vi "cluster_v9.vi"() -> ()   [LabVIEW 2009]
panel:
  out "Mixed Signal Graph":cluster{dbl[], dbl[], dbl[], dbl[], dbl[]}(graph)={[0.0, 0.004230646640570575, 0.00846129328114115, 0.012691939921711725, 0.0169225865622823, 0.021153233202852877, 0.02538387984342345, 0.029614526483994028, 0.0338451731245646, 0.038075819765135174, 0.042306466405705755, 0.04653711304627633, 0.0507677596868469, 0.054998406327417475, 0.059229052967988055, 0.06345969960855863, 0.0676903462491292, 0.07192099288969978, 0.07615163953027035, 0.08038228617084092, 0.08461293281141151, 0.08884357945198207, 0.09307422609255266, 0.09730487273312322, 0.1015355193736938, 0.10576616601426438, 0.10999681265483495, 0.11422745929540552, 0.11845810593597611, 0.12268875257654667, 0.12691939921711726, 0.13115004585768783, 0.1353806924982584, 0.13961133913882898, 0.14384198577939955, 0.14807263241997012, 0.1523032790605407, 0.15653392570111127, 0.16076457234168184, 0.16499521898225245, 0.16922586562282302, 0.17345651226339356, 0.17768715890396414, 0.18191780554453474, 0.1861484521851053, 0.19037909882567586, 0.19460974546624643, 0.19884039210681703, 0.2030710387473876, 0.2073016853879582, 0.21153233202852875, 0.21576297866909933, 0.2199936253096699, 0.2242242719502405, 0.22845491859081105, 0.23268556523138162, 0.23691621187195222, 0.2411468585125228, 0.24537750515309334, 0.2496081517936639, 0.2538387984342345, 0.2580694450748051, 0.26230009171537566, 0.2665307383559462, 0.2707613849965168, 0.2749920316370874, 0.27922267827765795, 0.2834533249182285, 0.2876839715587991, 0.2919146181993697, 0.29614526483994025, 0.3003759114805108, 0.3046065581210814, 0.308837204761652, 0.31306785140222254, 0.3172984980427931, 0.3215291446833637, 0.3257597913239343, 0.3299904379645049, 0.33422108460507544, 0.33845173124564604, 0.34268237788621664, 0.34691302452678713, 0.35114367116735773, 0.3553743178079283, 0.3596049644484989, 0.3638356110890695, 0.36806625772964, 0.3722969043702106, 0.3765275510107812, 0.3807581976513517, 0.3849888442919223, 0.38921949093249286, 0.39345013757306346, 0.39768078421363406, 0.40191143085420467, 0.4061420774947752, 0.4103727241353458, 0.4146033707759164, 0.4188340174164869, 0.4230646640570575, 0.42729531069762805, 0.43152595733819865, 0.43575660397876925, 0.4399872506193398, 0.4442178972599104, 0.448448543900481, 0.4526791905410515, 0.4569098371816221, 0.46114048382219264, 0.46537113046276324, 0.46960177710333384, 0.47383242374390444, 0.478063070384475, 0.4822937170250456, 0.4865243636656162, 0.4907550103061867, 0.4949856569467573, 0.4992163035873278, 0.5034469502278984], [0.0, 0.4105568446600889, 0.7487202054388066, 0.9548617406674794, 0.9926325157175458, 0.8553724102418765, 0.5672844971219748, 0.1791673148942777, -0.24054243798854055, -0.6178373454393544, -0.8861890005972879, -0.998278959074209, -0.9343423997307195, -0.7056532553692195, -0.35253628028746176, 0.06274341320109471, 0.4669595613333527, 0.7888367351766151, 0.9716183362245395, 0.9830744867844777, 0.8211851239548108, 0.5144961972940673, 0.11708616185075667, -0.30096967521764056, -0.6659555327812795, -0.9135134586098452, -0.9999915663780399, -0.9101411722988674, -0.6598055953672661, -0.29312650509683696, 0.12523957857763632, 0.5215221687456819, 0.8258447606627524, 0.9845461550595324, 0.9696425368160321, 0.7837618607724106, 0.45968046448105704, 0.05454361696822202, -0.3602109059217929, -0.7114494437517302, -0.9372381090279818, -0.9977635888978398, -0.882353426164791, -0.6113578935480203, -0.23256163031875554, 0.1872422226143023, 0.5740296565032156, 0.8595984474051875, 0.9935942535766267, 0.9523895959962669, 0.743250091479855, 0.40305330654732185, -0.008213863474088874, -0.4180326830398945, -0.7541398042254394, -0.9572694620667934, -0.99160380624181, -0.8510886622215772, -0.560501063798189, -0.17108031899001463, 0.24850701657486107, 0.6242751126536321, 0.8899647850177782, 0.99872697667578, 0.931383651574637, 0.6998094574851441, 0.3448378694917055, -0.07093897621799697, -0.4742071530352126, -0.793858387798745, -0.9735285818155787, -0.9815364917604706, -0.816470082961343, -0.507435513457404, -0.10892484547378199, 0.30879253930837325, 0.6720605390471127, 0.9168241113633988, 0.9999240982558683, 0.9067074799542068, 0.6536111417333007, 0.28526355811438003, -0.13338454555406226, -0.5285129537791516, -0.8304486787055756, -0.9859513972941013, -0.9676013168946559, -0.7786341069812652, -0.4523703535894608, -0.04634014074889865, 0.36786122859775133, 0.71719763157143, 0.940070584096705, 0.9971809009180234, 0.8784583205014747, 0.6048371941397673, 0.22456513202015538, -0.19530449734663968, -0.5807360868548394, -0.8637664885863127, -0.9944889549318572, -0.9498531948455234, -0.7377298314100129, -0.3955225749554867, 0.016427172769559645, 0.4254803173017054, 0.7595085221865201, 0.9596125977483974, 0.9905081945551012, 0.8467474923631642, 0.5536798142012235, 0.16298178052054185, -0.2564548287180254, -0.6306707608431243, -0.8936805246790326, -0.9991076114753917, -0.9283620641825999, -0.6939184443729015, -0.3371161929362305, 0.07912975307502212], [0.0, 0.0, 0.0, 0.0, 0.0, 0.0, 0.0, 0.0, 0.0, 0.0, 0.0, 0.0, 0.0, 0.0, 0.0, 0.0, 0.0, 0.0, 0.0, 0.0, 0.0, 0.0, 0.0, 0.0, 0.0, 0.0, 0.0, 0.0, 0.0, 0.0, 0.0, 0.0, 0.0, 0.0, 0.0, 0.0, 0.0, 0.0, 0.0, 0.0, 0.0, 0.0, 0.0, 0.0, 0.0, 0.0, 0.0, 0.0, 0.0, 0.0, 0.0, 0.0, 0.0, 0.0, 0.0, 0.0, 0.0, 0.0, 0.0, 0.0, 0.0, 0.0, 0.0, 0.0, 0.0, 0.0, 0.0, 0.0, 0.0, 0.0, 0.0, 0.0, 0.0, 0.0, 0.0, 0.0, 0.0, 0.0, 0.0, 0.0, 0.0, 0.0, 0.0, 0.0, 0.0, 0.0, 0.0, 0.0, 0.0, 0.0, 0.0, 0.0, 0.0, 0.0, 0.0, 0.0, 0.0, 0.0, 0.0, 0.0, 0.0, 0.0, 0.0, 0.0, 0.0, 0.0, 0.0, 0.0, 0.0, 0.0, 0.0, 0.0, 0.0, 0.0, 0.0, 0.0, 0.0, 0.0, 0.0, 0.0], [1.0, 0.9982936638442269, 0.9931804785430605, 0.9846778937224019, 0.9728149259180452, 0.957632059551749, 0.9391811087711717, 0.9175250406251635, 0.8927377601778635, 0.8649038582949328, 0.8341183229626493, 0.8004862151250378, 0.7641223101452946, 0.7251507061150838, 0.683704400348416, 0.6399248355053966, 0.5939614168947772, 0.5459710026025942, 0.49611736818692226, 0.44457064776556143, 0.39150675340404506, 0.33710677478540313, 0.2815563612104166, 0.2250450880373876, 0.16776580972356367, 0.10991400167607222, 0.051687093158409365, -0.006716206470939284, -0.06509658588842593, -0.12325481198967517, -0.1809924098067822, -0.2381123398383418, -0.29441967048069734, -0.3497222432656289, -0.40383132863423615, -0.45656227000907845, -0.5077351139665637, -0.5571752243590158, -0.6047138782906183, -0.6501888419133702, -0.6934449240780485, -0.7343345059507433, -0.772718044787567, -0.8084645501483116, -0.8414520309238988, -0.8715679116520576, -0.898709416700489, -0.9227839210064208, -0.943709266175594, -0.96141404086194, -0.9758378244711048, -0.9869313933561374, -0.9946568888016678, -0.998987946223296, -0.9999097851412794, -0.997419259621467, -0.9915248690113416, -0.9822467289345315, -0.9696165026427797, -0.9536772929596405, -0.9344834951846677, -0.9121006114600809, -0.88660502723342, -0.8580837505790422, -0.8266341152680752, -0.7923634486001533, -0.7553887051305126, -0.7158360675424179, -0.6738405160270151, -0.6295453676401688, -0.5831017872083147, -0.5346682714524423, -0.48441010809072127, -0.43249881176568583, -0.379111538720961, -0.3244304822250554, -0.2686422508054387, -0.21193723141478688, -0.15450893970270088, -0.09655335961020424, -0.03826827454077909, 0.020147407609582023, 0.07849433325984448, 0.1365733834723778, 0.19418635348064073, 0.2511366290970993, 0.30722985769302397, 0.36227461146031936, 0.41608304069190793, 0.46847151485122324, 0.5192612492430576, 0.5682789151471406, 0.6153572313322662, 0.6603355349323142, 0.7030603297359688, 0.7433858100189867, 0.7811743581313565, 0.8162970141412415, 0.8486339159329682, 0.878074708257152, 0.9045189193369975, 0.9278763037455517, 0.9480671503837738, 0.9650225545083945, 0.9786846528812267, 0.9890068212374359, 0.9959538333988778, 0.9995019814895009, 0.9996391568425592, 0.9963648913235233, 0.989690358927671, 0.9796383376469019, 0.9662431317359161, 0.9495504546430333, 0.929617273005174, 0.9065116122393948, 0.8803123243944311, 0.8511088190544934, 0.8190007582136563, 0.7840977161621274], [0.0, 0.0005842639199106157, 0.0011685278398212314, 0.0017527917597318472, 0.0023370556796424627, 0.002921319599553078, 0.0035055835194636943, 0.004089847439374309, 0.0046741113592849255, 0.005258375279195541, 0.005842639199106156, 0.0064269031190167724, 0.007011167038927389, 0.007595430958838004, 0.008179694878748619, 0.008763958798659235, 0.009348222718569851, 0.009932486638480467, 0.010516750558391082, 0.011101014478301698, 0.011685278398212312, 0.01226954231812293, 0.012853806238033545, 0.01343807015794416, 0.014022334077854777, 0.014606597997765392, 0.015190861917676008, 0.015775125837586623, 0.016359389757497237, 0.016943653677407855, 0.01752791759731847, 0.018112181517229087, 0.018696445437139702, 0.019280709357050316, 0.019864973276960934, 0.02044923719687155, 0.021033501116782163, 0.02161776503669278, 0.022202028956603396, 0.02278629287651401, 0.023370556796424625, 0.023954820716335243, 0.02453908463624586, 0.025123348556156472, 0.02570761247606709, 0.026291876395977708, 0.02687614031588832, 0.027460404235798937, 0.028044668155709555, 0.028628932075620166, 0.029213195995530784, 0.0297974599154414, 0.030381723835352016, 0.03096598775526263, 0.031550251675173245, 0.032134515595083867, 0.032718779514994474, 0.033303043434905095, 0.03388730735481571, 0.034471571274726324, 0.03505583519463694, 0.035640099114547553, 0.036224363034458175, 0.03680862695436879, 0.037392890874279404, 0.03797715479419002, 0.03856141871410063, 0.03914568263401125, 0.03972994655392187, 0.04031421047383248, 0.0408984743937431, 0.041482738313653705, 0.04206700223356433, 0.04265126615347494, 0.04323553007338556, 0.04381979399329618, 0.04440405791320679, 0.04498832183311741, 0.04557258575302802, 0.046156849672938635, 0.04674111359284925, 0.04732537751275987, 0.047909641432670486, 0.04849390535258111, 0.04907816927249172, 0.04966243319240233, 0.050246697112312944, 0.050830961032223565, 0.05141522495213418, 0.051999488872044794, 0.052583752791955415, 0.05316801671186602, 0.05375228063177664, 0.05433654455168726, 0.05492080847159787, 0.05550507239150849, 0.05608933631141911, 0.056673600231329724, 0.05725786415124033, 0.057842128071150946, 0.05842639199106157, 0.05901065591097218, 0.0595949198308828, 0.06017918375079342, 0.06076344767070403, 0.06134771159061464, 0.06193197551052526, 0.06251623943043588, 0.06310050335034649, 0.06368476727025711, 0.06426903119016773, 0.06485329511007834, 0.06543755902998895, 0.06602182294989957, 0.06660608686981019, 0.0671903507897208, 0.06777461470963142, 0.06835887862954204, 0.06894314254945265, 0.06952740646936326]}
  in  "Nr de perioade cosinus":dbl(knob)=1.1158618910882607 scale=0.0..25.0
  in  "stop":bool
  in  "Nr de perioade sinus":dbl(knob)=8.079939903863137 scale=0.0..25.0
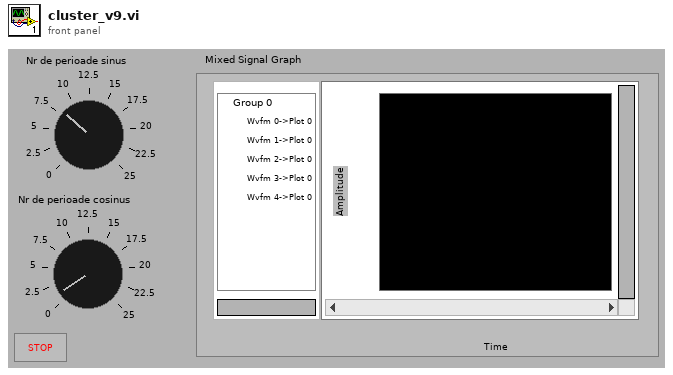
[diagram p1: front panel]
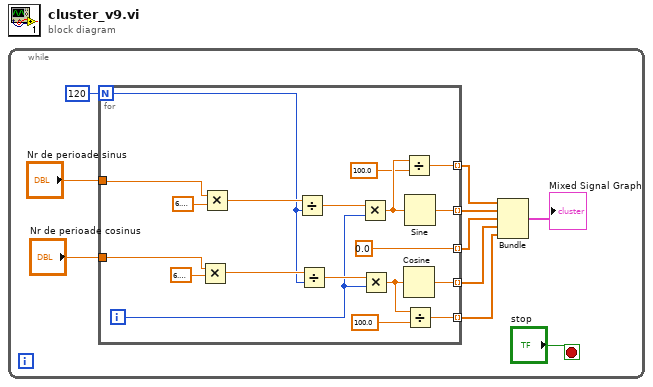
[diagram p0: block diagram]
diagram:
  n1 = while {
    stop <- "stop" stop-if-true
    n2 = for {
      N: 120 -> [w21]
      tunnel: [w29] -> w6 mode=indexing
      tunnel: "Nr de perioade sinus" -> [w26]
      tunnel: "Nr de perioade cosinus" -> [w23]
      tunnel: [w18] -> w1 mode=indexing
      tunnel: [w17] -> w5 mode=indexing
      tunnel: [w12] -> w3 mode=indexing
      tunnel: [0.0 ("y")] -> w2 mode=indexing
      i -> [w19]
      n3 = Multiply(x=w23, y=6.283185307179586) -> (x*y=w22:dbl)
      n4 = Multiply(x=w26, y=6.283185307179586) -> (x*y=w27:dbl)
      n5 = Divide(x=w27, y=w21) -> (x/y=w28:dbl)
      n6 = Divide(x=w22, y=w21) -> (x/y=w20:dbl)
      n7 = Multiply(x=w28, y=w19) -> (x*y=w16:dbl)
      n8 = Multiply(x=w20, y=w19) -> (x*y=w13:dbl)
      n9 = Divide(x=w16, y=100.0) -> (x/y=w17:dbl)
      n10 = Cosine(x=w13) -> (cos(x)=w18:dbl)
      n11 = Sine(x=w16) -> (sin(x)=w29:dbl)
      n12 = Divide(x=w13, y=100.0) -> (x/y=w12:dbl)
    }
    n13 = Bundle(w5, w6, w2, w1, w3) -> (→"Mixed Signal Graph":cluster{dbl[], dbl[], dbl[], dbl[], dbl[]})  [unwired: 1 in]
  }
